vi "B軸回home_function2.vi"(7 "A¶b Home_action":T1, 8 "error in (no error)":errorcluster) -> (0 "error out":errorcluster)   [LabVIEW 2014]
uses:
  axis motion function.ctl
  global/Global.vi
panel:
  out "error_code":u32
  out "state":u8
  # "A軸是彈簧的夾爪"
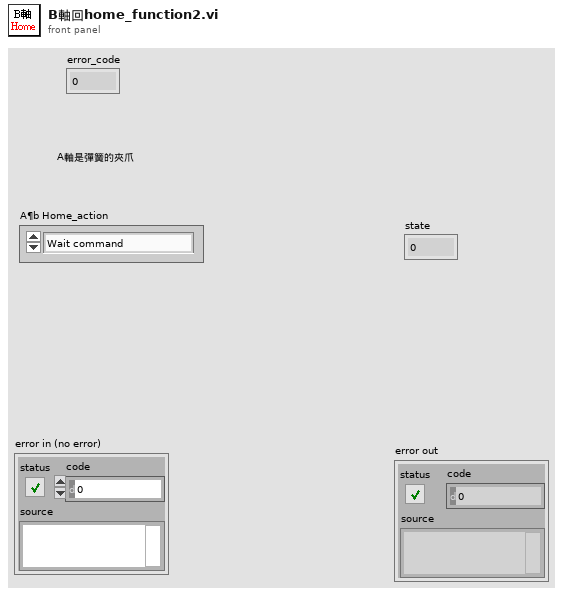
[diagram p1: front panel]
types:
  T1 = typedef "A¶b home_action.ctl" = enum16{"Wait command", "Config phi motor", "Start phi homing", "確認 phi homing done", "error"}
  T2 = typedef "axis motion function.ctl" = enum16{"Wait command", "Axis_S motion", "Axis_P motion", "Axis_Motion_Satus_CK", "Axis _S position CK", "Axis_P position CK", "finish", "error"}
  T3 = typedef "home function.ctl" = enum16{"Wait command", "Config X home mode_7", "Start X homing_7", "確認 X homing_7 done", "Config Y home mode_7", "Start Y homing_7", "確認 Y homing_7 done", "Config Z home mode_7", "Start Z homing_7", "確認 Z homing_7 done", "Config phi motor", "Start phi homing", "確認 phi homing done", "finish", "error"}
  T4 = typedef "軸參數記錄.ctl" = cluster{"X軸取料位":dbl, "X¶bCCD¦ì":dbl, "X軸影像異常排料位":dbl, "X軸迴轉缸位":dbl, "裝完料區已可安全取料位":dbl, "A軸取料角":dbl, "A¶bCCD¨¤":dbl, "B軸取料角":dbl, "B¶bCCD¨¤":dbl, "軸控參數PATH":path, "CCD左連續失敗報警次數":u8, "CCD右連續失敗報警次數":u8, "連續組裝失敗報警次數":u8, "ABVL/VH":i32, "XVL/VH":i32, "AB加速度":i32, "X加速度":i32, "home-XVL/VH":i32, "home-ABVL/VH":i32}
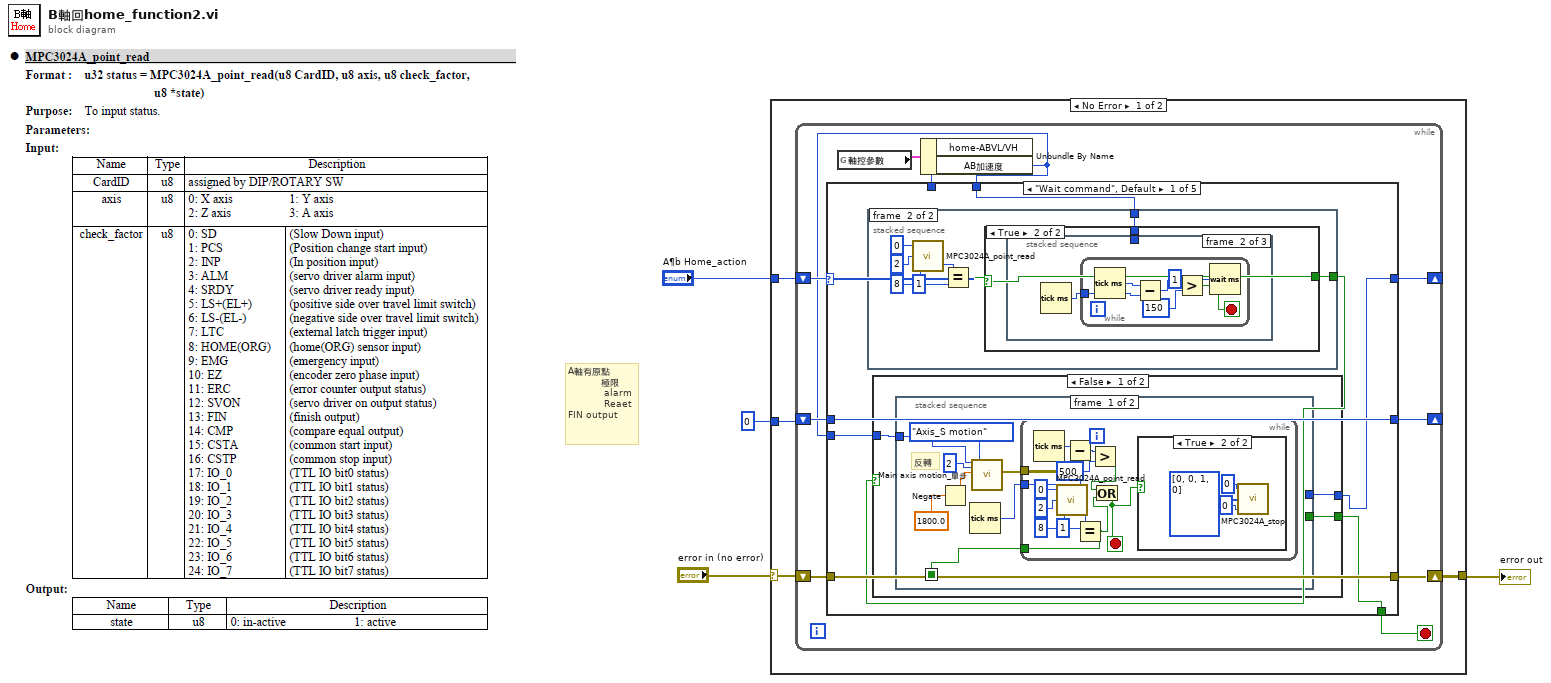
[diagram p0: block diagram]
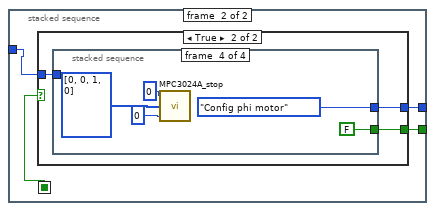
[diagram p3: hidden frame]
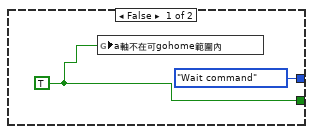
[diagram p4: hidden frame]
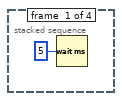
[diagram p5: hidden frame]
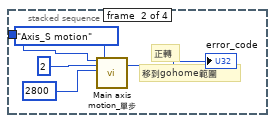
[diagram p6: hidden frame]
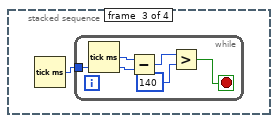
[diagram p7: hidden frame]
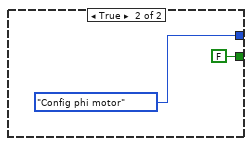
[diagram p8: hidden frame]
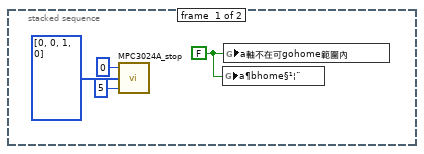
[diagram p9: hidden frame]
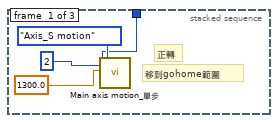
[diagram p11: hidden frame]
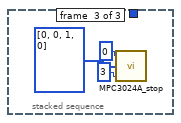
[diagram p12: hidden frame]
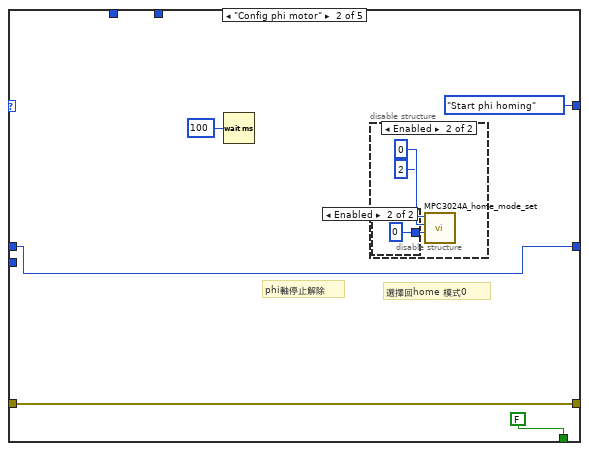
[diagram p13: hidden frame]
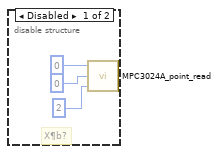
[diagram p14: hidden frame]
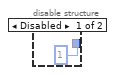
[diagram p15: hidden frame]
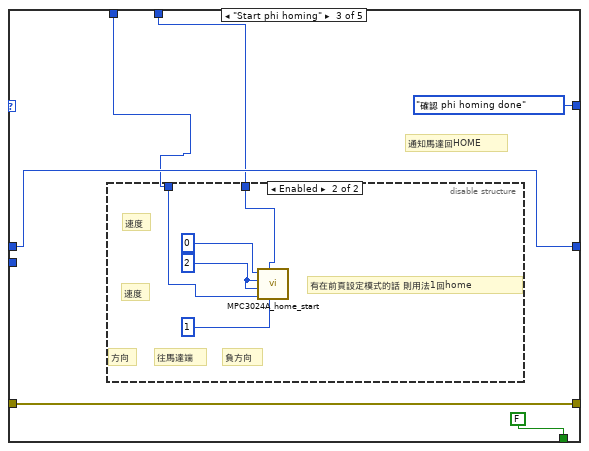
[diagram p16: hidden frame]
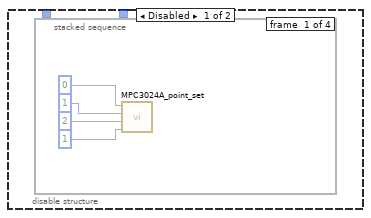
[diagram p17: hidden frame]
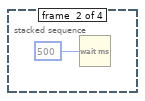
[diagram p18: hidden frame]
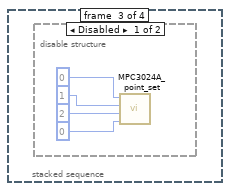
[diagram p19: hidden frame]
diagram:
  # "A軸有原點\n           極限\n            alarm\n            Reaet\nFIN output"
  n1 = case shown="No Error" "error in (no error)" {
    selector: "error in (no error)" -> [w7 w199]
    tunnel: [w6 w199] -> w3
    tunnel: "A¶b Home_action" -> [w8 _]
    tunnel: 0 -> [w5 _]
    frame No Error {
      n2 = while {
        shift-right: [w17] -> _
        shift-left: w8 -> [w18]
        shift-right: [w14] -> w6
        shift-left: w7 -> [w15]
        shift-right: [w12] -> _
        shift-left: w5 -> [w13]
        stop <- w16 stop-if-true
        n3 = global read "Global.vi" "軸控參數"() -> (w11:T4)
        n4 = Unbundle By Name(w11) -> ("home-ABVL/VH"=w10:i32, "AB加速度"=w9:i32)
        n5 = case shown="\"Wait command\", Default" w18 {
          tunnel: [w22 A¶b_home_action."Start phi homing" ("A¶b Home_action") A¶b_home_action."確認 phi homing done" ("A¶b Home_action") w146 _] -> w17
          tunnel: [w21 FALSE FALSE w147 TRUE] -> w16
          tunnel: w15 -> [w25 w110 w126 _ w191]
          tunnel: [w25 w110 w126 w148 w191] -> w14
          tunnel: w13 -> [w24 w109 w124 w150 w192]
          tunnel: [w24 w109 w124 w149 w192] -> w12
          tunnel: w10 -> [_ _ w123 _ _]
          tunnel: w9 -> [w20 _ w122 _ _]
          tunnel: w9 -> [w19 _ _ _ _]
          frame "Wait command", Default {
            n6 = stacked-sequence {
              tunnel: [_ w85] -> w23
              tunnel: w20 -> [_ w84]
              frame #0 {
                w80 = FALSE ("a軸不在可gohome範圍內")
                n7 = call "MPC3024A_stop.vi"("Tdec_ms"=u32 5, "axis[4]"=u8[] [0, 0, 1, 0], "CardID"=u8 0) -> ()  [unwired: 1 out]
                n8 = global write "Global.vi" "a¶bhome§¹¦¨"(w80) -> ()
                n9 = global write "Global.vi" "a軸不在可gohome範圍內"(w80) -> ()
              }
              frame #1 {
                n10 = call "MPC3024A_point_read.vi"("check_factor"=u8 8, "axis"=u8 2, "CardID"=u8 0) -> ("state"=w88:u8)  [unwired: 1 out]
                n11 = Equal?(x=w88, y=u8 1) -> (x = y?=w86:bool)
                n12 = case shown="True" w86 {
                  selector: w86 -> [w92 w94]
                  tunnel: [w92 w94] -> w85
                  tunnel: w84 -> [_ w93]
                  frame False {
                  }
                  frame True {
                    n13 = stacked-sequence {
                      tunnel: w93 -> [w95 _ _]
                      frame #0 {
                        # "移到gohome範圍"
                        # "正轉"
                        n14 = call "Main axis motion_單步.vi"("Tacc/Tdec"=w95, "axis"=u8 2, "VL/VH"=1300.0 ("轉速(rpm)"), "Axis motion function"=axis_motion_function."Axis_S motion") -> ()  [unwired: 13 in, 3 out]
                      }
                      frame #1 {
                        n15 = Tick Count (ms)() -> (millisecond timer value=w99:u32)
                        n16 = while {
                          tunnel: w99 -> [w104]
                          stop <- w101 stop-if-true
                          n17 = Tick Count (ms)() -> (millisecond timer value=w105:u32)
                          n18 = Subtract(x=w105, y=w104) -> (x-y=w103:u32)
                          n19 = Greater?(x=w103, y=u32 150) -> (0:w101:bool)
                          n20 = Wait (ms)(milliseconds to wait=u32 1) -> ()  [unwired: 1 out]
                        }
                      }
                      frame #2 {
                        n21 = call "MPC3024A_stop.vi"("Tdec_ms"=u32 3, "axis[4]"=u8[] [0, 0, 1, 0], "CardID"=u8 0) -> ()  [unwired: 1 out]
                      }
                    }
                  }
                }
              }
            }
            n22 = case shown="False" w23 {
              tunnel: [w28 A¶b_home_action."Config phi motor" ("A¶b Home_action")] -> w22
              tunnel: [w27 FALSE] -> w21
              tunnel: w19 -> [w26 _]
              frame False {
                n23 = stacked-sequence {
                  seq-local: [w31 _] -> [_ w55]
                  tunnel: [_ w54] -> w28
                  tunnel: [_ w53] -> w27
                  tunnel: w26 -> [w29 w52]
                  frame #0 {
                    # "反轉"
                    n24 = Negate(x=1800.0 ("轉速(rpm)")) -> (-x=w36:dbl)
                    n25 = Tick Count (ms)() -> (millisecond timer value=w33:u32)
                    n26 = call "Main axis motion_單步.vi"("Tacc/Tdec"=w29, "axis"=u8 2, "VL/VH"=w36, "Axis motion function"=axis_motion_function."Axis_S motion") -> ("error out"=w32:errorcluster)  [unwired: 13 in, 2 out]
                    n27 = while {
                      tunnel: w33 -> [w47]
                      tunnel: w32 -> [_]
                      tunnel: [w37] -> w31
                      stop <- w38 stop-if-true
                      n28 = Tick Count (ms)() -> (millisecond timer value=w48:u32)
                      n29 = call "MPC3024A_point_read.vi"("check_factor"=u8 8, "axis"=u8 2, "CardID"=u8 0) -> ("state"=w43:u8)  [unwired: 1 out]
                      n30 = Subtract(x=w48, y=w47) -> (x-y=w46:u32)
                      n31 = Equal?(x=w43, y=u8 1) -> (x = y?=w37:bool)
                      n32 = Greater?(x=w46, y=u32 500) -> (0:w39:bool)
                      n33 = Or(x=w39, y=w37) -> (x .or. y?=w38:bool)
                      n34 = case shown="True" w38 {
                        frame False {
                        }
                        frame True {
                          n35 = call "MPC3024A_stop.vi"("Tdec_ms"=u32 0, "axis[4]"=u8[] [0, 0, 1, 0], "CardID"=u8 0) -> ()  [unwired: 1 out]
                        }
                      }
                    }
                  }
                  frame #1 {
                    n36 = case shown="True" w55 {
                      tunnel: [A¶b_home_action."Wait command" ("A¶b Home_action") w60] -> w54
                      tunnel: [w56 w59] -> w53
                      tunnel: w52 -> [_ w58]
                      frame False {
                        w56 = TRUE
                        n37 = global write "Global.vi" "a軸不在可gohome範圍內"(w56) -> ()
                      }
                      frame True {
                        n38 = stacked-sequence {
                          tunnel: [_ _ _ A¶b_home_action."Config phi motor" ("A¶b Home_action")] -> w60
                          tunnel: [_ _ _ FALSE] -> w59
                          tunnel: w58 -> [_ w63 _ _]
                          frame #0 {
                            n39 = Wait (ms)(milliseconds to wait=u32 5) -> ()  [unwired: 1 out]
                          }
                          frame #1 {
                            # "移到gohome範圍"
                            # "正轉"
                            n40 = call "Main axis motion_單步.vi"("Tacc/Tdec"=w63, "axis"=u8 2, "VL/VH"=2800, "Axis motion function"=axis_motion_function."Axis_S motion") -> ("error_code"=→"error_code":u32)  [unwired: 13 in, 2 out]
                          }
                          frame #2 {
                            n41 = Tick Count (ms)() -> (millisecond timer value=w67:u32)
                            n42 = while {
                              tunnel: w67 -> [w71]
                              stop <- w68 stop-if-true
                              n43 = Tick Count (ms)() -> (millisecond timer value=w72:u32)
                              n44 = Subtract(x=w72, y=w71) -> (x-y=w70:u32)
                              n45 = Greater?(x=w70, y=u32 140) -> (0:w68:bool)
                            }
                          }
                          frame #3 {
                            n46 = call "MPC3024A_stop.vi"("Tdec_ms"=u32 0, "axis[4]"=u8[] [0, 0, 1, 0], "CardID"=u8 0) -> ()  [unwired: 1 out]
                          }
                        }
                      }
                    }
                  }
                }
              }
              frame True {
              }
            }
          }
          frame "Config phi motor" {
            # "選擇回home 模式0"
            # "phi軸停止解除"
            n47 = Wait (ms)(milliseconds to wait=u32 100) -> ()  [unwired: 1 out]
            n48 = disable-structure shown="Enabled" {
              frame Disabled {
                # "X¶b?"
                n49 = call "MPC3024A_point_read.vi"("check_factor"=u8 2, "axis"=u8 0, "CardID"=u8 0) -> ()  [unwired: 2 out]
              }
              frame Enabled {
                n50 = disable-structure shown="Enabled" {
                  disable-tunnel: [u8 1 ("mode") u8 0 ("mode")] -> w117
                  frame Disabled {
                  }
                  frame Enabled {
                  }
                }
                n51 = call "MPC3024A_home_mode_set.vi"("mode"=w117, "axis"=u8 2, "CardID"=u8 0) -> ()  [unwired: 1 in, 1 out]
              }
            }
          }
          frame "Start phi homing" {
            # "通知馬達回HOME"
            n52 = disable-structure shown="Enabled" {
              disable-tunnel: w123 -> [_ w143]
              disable-tunnel: w122 -> [_ w141]
              frame Disabled {
                n53 = stacked-sequence {
                  frame #0 {
                    n54 = call "MPC3024A_point_set.vi"("on_off"=u8 1, "check_factor"=u8 2, "axis"=u8 1, "CardID"=u8 0) -> ()  [unwired: 1 out]
                  }
                  frame #1 {
                    n55 = Wait (ms)(milliseconds to wait=u32 500) -> ()  [unwired: 1 out]
                  }
                  frame #2 {
                    n56 = disable-structure shown="Disabled" {
                      frame Disabled {
                        n57 = call "MPC3024A_point_set.vi"("on_off"=u8 0, "check_factor"=u8 2, "axis"=u8 1, "CardID"=u8 0) -> ()  [unwired: 1 out]
                      }
                      frame Enabled {
                      }
                    }
                  }
                  frame #3 {
                    n58 = disable-structure shown="Disabled" {
                      frame Disabled {
                        n59 = call "MPC3024A_point_read.vi"("check_factor"=u8 8, "axis"=u8 1, "CardID"=u8 0) -> ("state"=→"state":u8)  [unwired: 1 out]
                      }
                      frame Enabled {
                      }
                    }
                  }
                }
              }
              frame Enabled {
                w142 = u8 2 ("axis")
                # "負方向"
                # "往馬達端"
                # "有在前頁設定模式的話 則用法1回home"
                # "速度"
                # "速度"
                # "方向"
                n60 = call "MPC3024A_home_start.vi"("direction"=u8 1, "Tacc_ms"=w141, "VH"=w143, "VL"=w142, "axis"=w142, "CardID"=u8 0) -> ()  [unwired: 1 out]
              }
            }
          }
          frame "確認 phi homing done" {
            n61 = disable-structure shown="Enabled" {
              disable-tunnel: [w154 w159] -> w152
              frame Disabled {
                n62 = call "MPC3024A_point_read.vi"("check_factor"=u8 8, "axis"=u8 1, "CardID"=u8 0) -> ("state"=w158:u8)  [unwired: 1 out]
                n63 = Equal?(x=w158, y=u8 1) -> (x = y?=w154:bool)
              }
              frame Enabled {
                n64 = call "MPC3024A_motion_status_read.vi"("check_factor"=u8 0, "axis"=u8 2, "CardID"=u8 0) -> ("ret_fig"=w160:u8)  [unwired: 1 out]
                n65 = Equal?(x=w160, y=u8 1) -> (x = y?=w159:bool)
              }
            }
            n66 = Wait (ms)(milliseconds to wait=u32 100) -> ()  [unwired: 1 out]
            n67 = case shown="True" w152 {
              selector: w152 -> [_ w180]
              tunnel: w150 -> [w173 _]
              tunnel: [w171 0] -> w149
              tunnel: [w169 errorcluster {"status"=FALSE, "code"=0, "source"=""} ("error in (no error)")] -> w148
              tunnel: [w166 w180] -> w147
              tunnel: [w165 _] -> w146
              frame False {
                n68 = Increment(x=w173) -> (x+1=w170:i32)
                n69 = Wait (ms)(milliseconds to wait=u32 100) -> ()  [unwired: 1 out]
                n70 = Less?(x=w170, y=100) -> (x < y?=w167:bool)
                n71 = Not(x=w167) -> (.not. x?=w166:bool)
                n72 = case shown="False" w167 {
                  tunnel: [0 w179] -> w171
                  tunnel: w170 -> [_ w179]
                  tunnel: [errorcluster {"status"=TRUE, "code"=0, "source"="B軸回home失敗"} ("error in (no error)") errorcluster {"status"=FALSE, "code"=0, "source"=""} ("error in (no error)")] -> w169
                  tunnel: [A¶b_home_action."error" ("A¶b Home_action") A¶b_home_action."確認 phi homing done" ("A¶b Home_action")] -> w165
                  frame False {
                  }
                  frame True {
                  }
                }
              }
              frame True {
                n73 = disable-structure shown="Enabled" {
                  frame Enabled {
                    n74 = call "MPC3024A_current_position_set.vi"("current_posi"=0, "axis"=u8 2, "CardID"=u8 0) -> ()  [unwired: 1 out]
                  }
                  frame Disabled {
                  }
                }
                n75 = global write "Global.vi" "a¶bhome§¹¦¨"(w180) -> ()
                n76 = disable-structure shown="Disabled" {
                  frame Disabled {
                    n77 = call "MPC3024A_FB_counter_set.vi"("value"=0, "axis"=u8 3, "CardID"=u8 0) -> ()  [unwired: 1 out]
                  }
                  frame Enabled {
                  }
                }
                n78 = disable-structure shown="Disabled" {
                  disable-tunnel: [home_function."finish" ("Home function") _] -> _
                  frame Disabled {
                  }
                  frame Enabled {
                  }
                }
              }
            }
          }
          frame "error" {
            n79 = disable-structure shown="Enabled" {
              frame Disabled {
                # "各軸STOP"
                n80 = call "MPC3024A_stop.vi"("Tdec_ms"=u32 10, "axis[4]"=u8[] [1, 1, 1, 1], "CardID"=u8 0) -> ()  [unwired: 1 out]
              }
              frame Enabled {
                n81 = call "MPC3024A_stop.vi"("Tdec_ms"=u32 10, "axis[4]"=u8[] [0, 0, 1, 0], "CardID"=u8 0) -> ()  [unwired: 1 out]
              }
            }
          }
        }
      }
    }
    frame Error {
    }
  }
  "error out" <- w3
